vi "ControlSub.vi"(0 "AxisForceSample":dbl[](array[numeric]), 1 "Command":dbl[](array[numeric]), 3 "Angel":bool[](array[boolean]), 4 "AngleSample":dbl[](array[numeric]), 5 "TorqueSample":dbl[](array[numeric]), 6 "Torque":bool[](array[boolean]), 7 "ControlPara":dbl[][](array[numeric]), 8 "syn-error":dbl[](array[numeric]), 11 "ChannelSetArray":T1[](array[typedef]) {"Enable" items=["不使能", "使能"]; "Wave" items=["0指令", "正弦波", "方波", "三角波", "常值", "波形数据", "白噪声", "正弦扫频", "梯度加载", "VMIC"]; "ChannelType" items=["标准波形跟踪"=1, "扫频测试"=2, "消除多余力"=3, "梯度加载"=4, "载荷谱跟踪"=5, "模拟输入跟踪"=9]; "ChannelStatus" items=["通道关", "位置通道", "加载通道"]}, 13 "dt":dbl=0.001) -> (9 "syn out":dbl[](array[numeric]), 10 "diff syn out 2":dbl[](array[numeric]), 14 "ControlOut":dbl[](array[numeric]), 15 "Forward":dbl[](array[numeric]), 18 "PIDcontrolOut":dbl[](array[numeric]), 19 "CommandOut":dbl[](array[numeric]))   [LabVIEW 2020]
uses:
  ChannelCommand.ctl
  Control 1.ctl
  WaveType.ctl
  MoterEnable.ctl
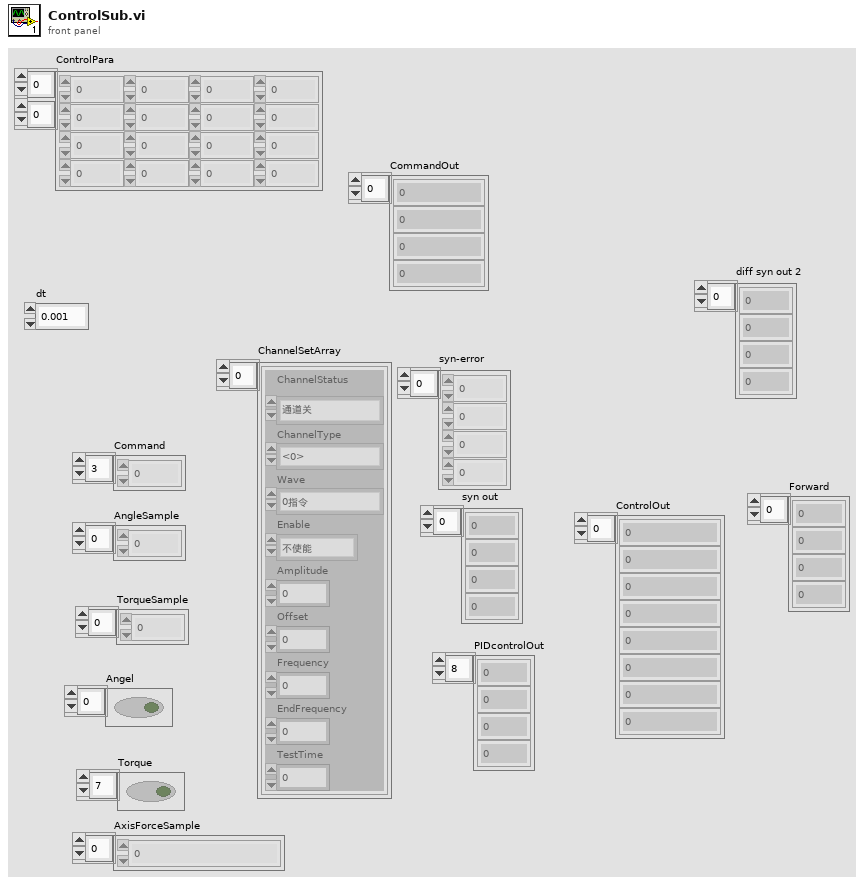
[diagram p1: front panel]
types:
  T1 = typedef "ChannelCommand.ctl" = cluster{"ChannelStatus":T2, "ChannelType":i32, "Wave":T3, "Enable":T4, "Amplitude":dbl, "Offset":dbl, "Frequency":dbl, "EndFrequency":dbl, "TestTime":dbl}
  T2 = typedef "Control 1.ctl" = i32
  T3 = typedef "WaveType.ctl" = i32
  T4 = typedef "MoterEnable.ctl" = u16
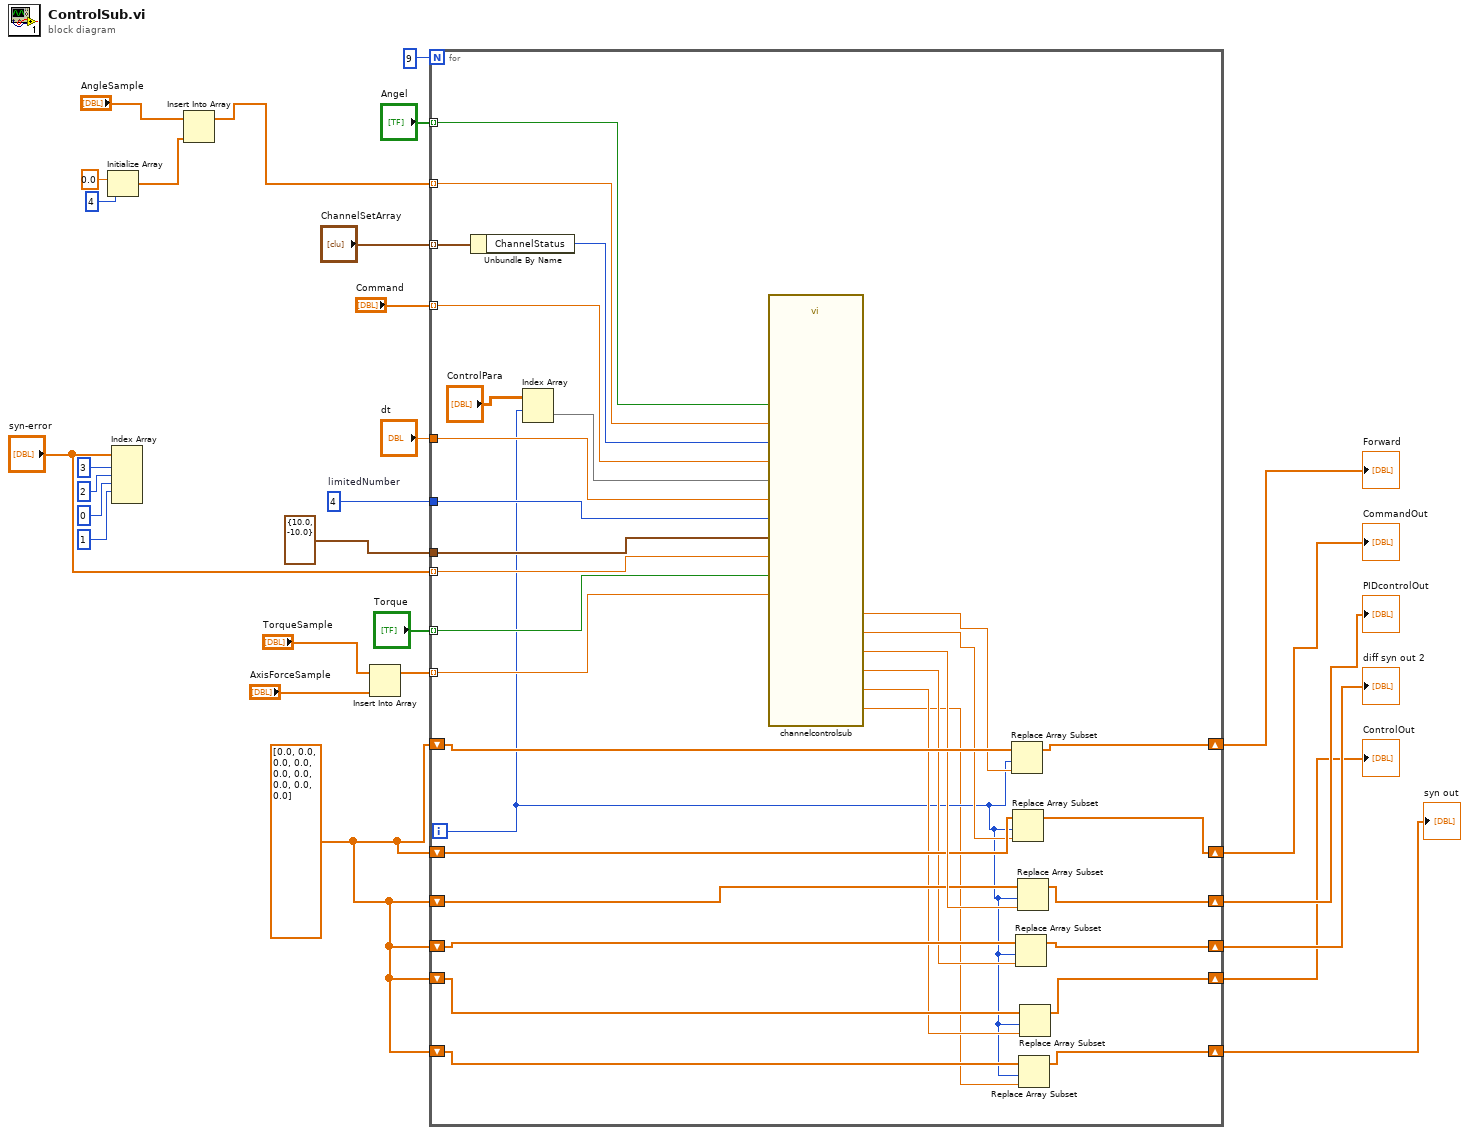
[diagram p0: block diagram]
diagram:
  w2 = dbl[] [0.0, 0.0, 0.0, 0.0, 0.0, 0.0, 0.0, 0.0, 0.0]
  w18 = 4  # limitedNumber
  n1 = Initialize Array(0.0 ("元素"), 4 ("维数大小")) -> (w10:dbl[])
  n2 = Index Array(array="syn-error", index #1=3 ("索引"), index #2=2 ("索引"), index #3=0 ("索引"), index #4=1 ("索引")) -> ()  [unwired: 1 in, 5 out]
  n3 = Insert Into Array(array="AngleSample", new element=w10) -> (w8:dbl[])  [unwired: 1 in]
  n4 = Insert Into Array(array="TorqueSample", new element="AxisForceSample") -> (w13:dbl[])  [unwired: 1 in]
  n5 = for {
    N: 9 -> [_]
    tunnel: "ChannelSetArray" -> [w60] mode=indexing
    tunnel: "Angel" -> [w58] mode=indexing
    tunnel: w8 -> [w57] mode=indexing
    tunnel: w13 -> [w56] mode=indexing
    tunnel: "Command" -> [w55] mode=indexing
    tunnel: "dt" -> [w54]
    tunnel: "syn-error" -> [w53] mode=indexing
    tunnel: "Torque" -> [w52] mode=indexing
    tunnel: w18 -> [w51]
    tunnel: cluster{"output high":dbl, "output low":dbl} {"output high"=10.0, "output low"=-10.0} ("output range") -> [w50]
    shift-right: [w45] -> w7
    shift-left: w2 -> [w47]
    shift-right: [w41] -> w5
    shift-left: w2 -> [w43]
    shift-right: [w40] -> w4
    shift-left: w2 -> [w42]
    shift-right: [w38] -> w3
    shift-left: w2 -> [w39]
    shift-right: [w36] -> w6
    shift-left: w2 -> [w37]
    shift-right: [w31] -> w1
    shift-left: w2 -> [w32]
    i -> [w30]
    n6 = Unbundle By Name(w60) -> ("ChannelStatus"=w59:T2)
    n7 = Index Array(array="ControlPara", index (row)=w30) -> (element=w48:dbl[])  [unwired: 1 in]
    n8 = call "channelcontrolsub.vi"("TorqueSample"=w56, "dt"=w54, "Limit Number"=w51, "Torque"=w52, "ControlPara"=w48, "AngleSample"=w57, "Angel"=w58, "syn-Error"=w53, "Command"=w55, "output range"=w50, "ChannelStatus"=w59) -> ("syn out"=w29:dbl, "ControlOut"=w33:dbl, "forward"=w46:dbl, "diff syn out 2"=w34:dbl, "PIDcontrol out"=w44:dbl, "Commandout"=w35:dbl)  [unwired: 11 in]
    n9 = Replace Array Subset(array=w47, new element=w46, index=w30) -> (w45:dbl[])
    n10 = Replace Array Subset(array=w37, new element=w35, index=w30) -> (w36:dbl[])
    n11 = Replace Array Subset(array=w42, new element=w34, index=w30) -> (w40:dbl[])
    n12 = Replace Array Subset(array=w43, new element=w44, index=w30) -> (w41:dbl[])
    n13 = Replace Array Subset(array=w32, new element=w29, index=w30) -> (w31:dbl[])
    n14 = Replace Array Subset(array=w39, new element=w33, index=w30) -> (w38:dbl[])
  }
  "ControlOut" <- w3
  "CommandOut" <- w6
  "syn out" <- w1
  "PIDcontrolOut" <- w5
  "Forward" <- w7
  "diff syn out 2" <- w4
